vi "Slow Mode.vi"(0 "Axes 4 Input":dbl, 1 "Axes 1 Input":dbl, 2 "Rotations Input":dbl, 3 "Boolean":bool) -> (4 "Axes 4 Output":dbl, 5 "Axes 1 Output":dbl, 6 "Rotations Output":dbl)   [LabVIEW 2014]
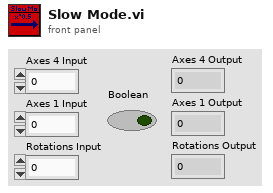
[diagram p1: front panel]
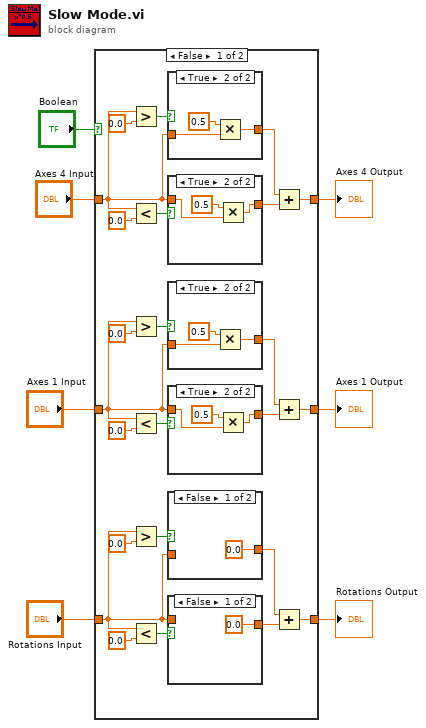
[diagram p0: block diagram]
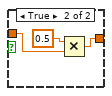
[diagram p2: hidden frame]
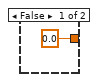
[diagram p3: hidden frame]
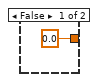
[diagram p4: hidden frame]
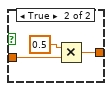
[diagram p5: hidden frame]
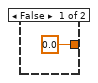
[diagram p6: hidden frame]
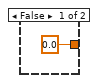
[diagram p7: hidden frame]
diagram:
  n1 = case shown="False" "Boolean" {
    tunnel: "Axes 4 Input" -> [w21 w56]
    tunnel: "Axes 1 Input" -> [w16 w57]
    tunnel: "Rotations Input" -> [w11 w58]
    tunnel: [w10 w58] -> w3
    tunnel: [w14 w57] -> w2
    tunnel: [w20 w56] -> w1
    frame False {
      n2 = Greater?(x=w21, y=0.0) -> (0:w29:bool)
      n3 = Less?(x=w21, y=0.0) -> (x < y?=w22:bool)
      n4 = Greater?(x=w16, y=0.0) -> (0:w25:bool)
      n5 = Less?(x=w16, y=0.0) -> (x < y?=w17:bool)
      n6 = Greater?(x=w11, y=0.0) -> (0:w24:bool)
      n7 = Less?(x=w11, y=0.0) -> (x < y?=w12:bool)
      n8 = case shown="True" w29 {
        tunnel: [0.0 ("y") w54] -> w19
        tunnel: w21 -> [_ w53]
        frame False {
        }
        frame True {
          n9 = Multiply(x=0.5 ("y"), y=w53) -> (x*y=w54:dbl)
        }
      }
      n10 = case shown="True" w22 {
        tunnel: [0.0 ("y") w42] -> w18
        tunnel: w21 -> [_ w41]
        frame False {
        }
        frame True {
          n11 = Multiply(x=0.5 ("y"), y=w41) -> (x*y=w42:dbl)
        }
      }
      n12 = case shown="True" w25 {
        tunnel: [0.0 ("y") w50] -> w15
        tunnel: w16 -> [_ w49]
        frame False {
        }
        frame True {
          n13 = Multiply(x=0.5 ("y"), y=w49) -> (x*y=w50:dbl)
        }
      }
      n14 = case shown="True" w17 {
        tunnel: [0.0 ("y") w38] -> w13
        tunnel: w16 -> [_ w37]
        frame False {
        }
        frame True {
          n15 = Multiply(x=0.5 ("y"), y=w37) -> (x*y=w38:dbl)
        }
      }
      n16 = case shown="False" w24 {
        tunnel: [0.0 ("y") w46] -> w9
        tunnel: w11 -> [_ w45]
        frame False {
        }
        frame True {
          n17 = Multiply(x=0.5 ("y"), y=w45) -> (x*y=w46:dbl)
        }
      }
      n18 = case shown="False" w12 {
        tunnel: [0.0 ("y") w34] -> w8
        tunnel: w11 -> [_ w33]
        frame False {
        }
        frame True {
          n19 = Multiply(x=0.5 ("y"), y=w33) -> (x*y=w34:dbl)
        }
      }
      n20 = Add(x=w19, y=w18) -> (x+y=w20:dbl)
      n21 = Add(x=w15, y=w13) -> (x+y=w14:dbl)
      n22 = Add(x=w9, y=w8) -> (x+y=w10:dbl)
    }
    frame True {
    }
  }
  "Axes 4 Output" <- w1
  "Axes 1 Output" <- w2
  "Rotations Output" <- w3
